vi "HSPA_PSK_TX.vi"() -> ()   [LabVIEW 2025]
doc: "This example shows how simple is to broadcast an Frequency Modulated sound signal using the USRP.\n\n1. Ask the user for a *.wav file.\n2. Read the WAV file.\n3. Select only one channel of the audio data.\n4. Modulate in FM using a frequency deviation of 75kHz. Similar to Radio FM.\n5. Initialize a session.\n6. Configure for arbitrary waveform mode.\n7. Set the output power level and center frequency.\n8. Set the IQ rate to 200k.\n9. Write and read the IQ rate to get the coerced value in order to resample our signal (if needed).\n10. Resample and write the signal to the on board memory. If resample is needed, this step will take little longer depending on the size of the file.\n11. Start the generation.\n12. Check for p the generation.\n13. Stop the generation.\n14. Close the session.\n15. Check for errors."
uses:
  <vilib>/addons/Modulation/Analog/support/mod_Set Error Source.vi
  <vilib>/addons/Modulation/Digital/General/MT Generate PSK System Parameters(M).vi
  Instance           1 28Saved   fm_sound_transmitter .vi
  <vilib>/sound2/lvsound2.llb/Sound File Info (path).vi
  <vilib>/sound2/lvsound2.llb/Sound File Read Open.vi
  <vilib>/addons/Modulation/Digital/Support/Common/Validators/mod_Generate Filter Coefficients Validate.vi
  <vilib>/addons/Modulation/Digital/General/subVIs/mod_Generate Filter Coefficients.vi
  <vilib>/sound2/lvsound2.llb/Sound File Read (DBL).vi
  <vilib>/Waveform/WDTOps.llb/WDT Index Channel DBL.vi
  <instrlib>/niUSRP/niUSRP Write Tx Data (CDB Cluster).vi
  <vilib>/addons/Modulation/niDMT.lvlib
  <vilib>/addons/Modulation/niAMT.lvlib
panel:
  out "sound Chart":waveform(dbl)[](graph)
  out "Frame Size [samples]":i32=4092
  in  "Enabled Channel":string(combo)="0"
  in  "Device Name":refnum<k15>="192.168.10.5"
  in  "filter parameter":dbl=0.5 format="%.2f"
  in  "pulse shaping samples per symbol (16)":i32=16
  in  "pulse shaping filter (none)":T1(ring)
  in  "M":i32=4 min=2 step=2
  in  "Select PSK Modulation Format":T2(tab)=enum."QPSK" caption="PSK"
  in  "QPSK System Parameters":T3={"Samples per Symbol"=8, "symbol map"=[], "Differential PSK"=enum."disable", "PSK type"=0} {"PSK type" items=["normal", "shifted", "offset"]; "symbol map" format="%.3f"}
  in  "pi/4 DQPSK System Parameters":T3={"Samples per Symbol"=8, "symbol map"=[], "Differential PSK"=enum."enable", "PSK type"=1} {"PSK type" items=["normal", "shifted", "offset"]; "symbol map" format="%.3f"}
  in  "OQPSK System Parameters":T3={"Samples per Symbol"=8, "symbol map"=[], "Differential PSK"=enum."disable", "PSK type"=2} {"PSK type" items=["normal", "shifted", "offset"]; "symbol map" format="%.3f"}
  in  "8-PSK System Parameters":T3={"Samples per Symbol"=8, "symbol map"=[], "Differential PSK"=enum."disable", "PSK type"=0} {"PSK type" items=["normal", "shifted", "offset"]; "symbol map" format="%.3f"}
  in  "16-PSK System Parameters":T3={"Samples per Symbol"=8, "symbol map"=[], "Differential PSK"=enum."disable", "PSK type"=0} {"PSK type" items=["normal", "shifted", "offset"]; "symbol map" format="%.3f"}
  in  "Custom System Parameters":T3={"Samples per Symbol"=8, "symbol map"=[], "Differential PSK"=enum."disable", "PSK type"=0} {"PSK type" items=["normal", "shifted", "offset"]; "symbol map" format="%.3f"}
  in  "BPSK System Parameters":T3={"Samples per Symbol"=8, "symbol map"=[], "Differential PSK"=enum."disable", "PSK type"=0} {"PSK type" items=["normal", "shifted", "offset"]; "symbol map" format="%.3f"}
  in  "IQ rate":dbl=100000.0 format="%#_6p"
  out "Constellation Graph 2":T4(graph)
  out "Waveform Graph":waveform(dbl)[](graph)
  in  "Transmitter Gain":dbl format="%.2f"
  in  "frequency (Hz)":dbl=94700000.0 min=500000.0 max=2700000000.0 format="%.2p"
  out "Status":string="Stopped"
  in  "stop":bool
  out "Audio Data":waveform(dbl)[](graph)
  # "USRP Configuration"
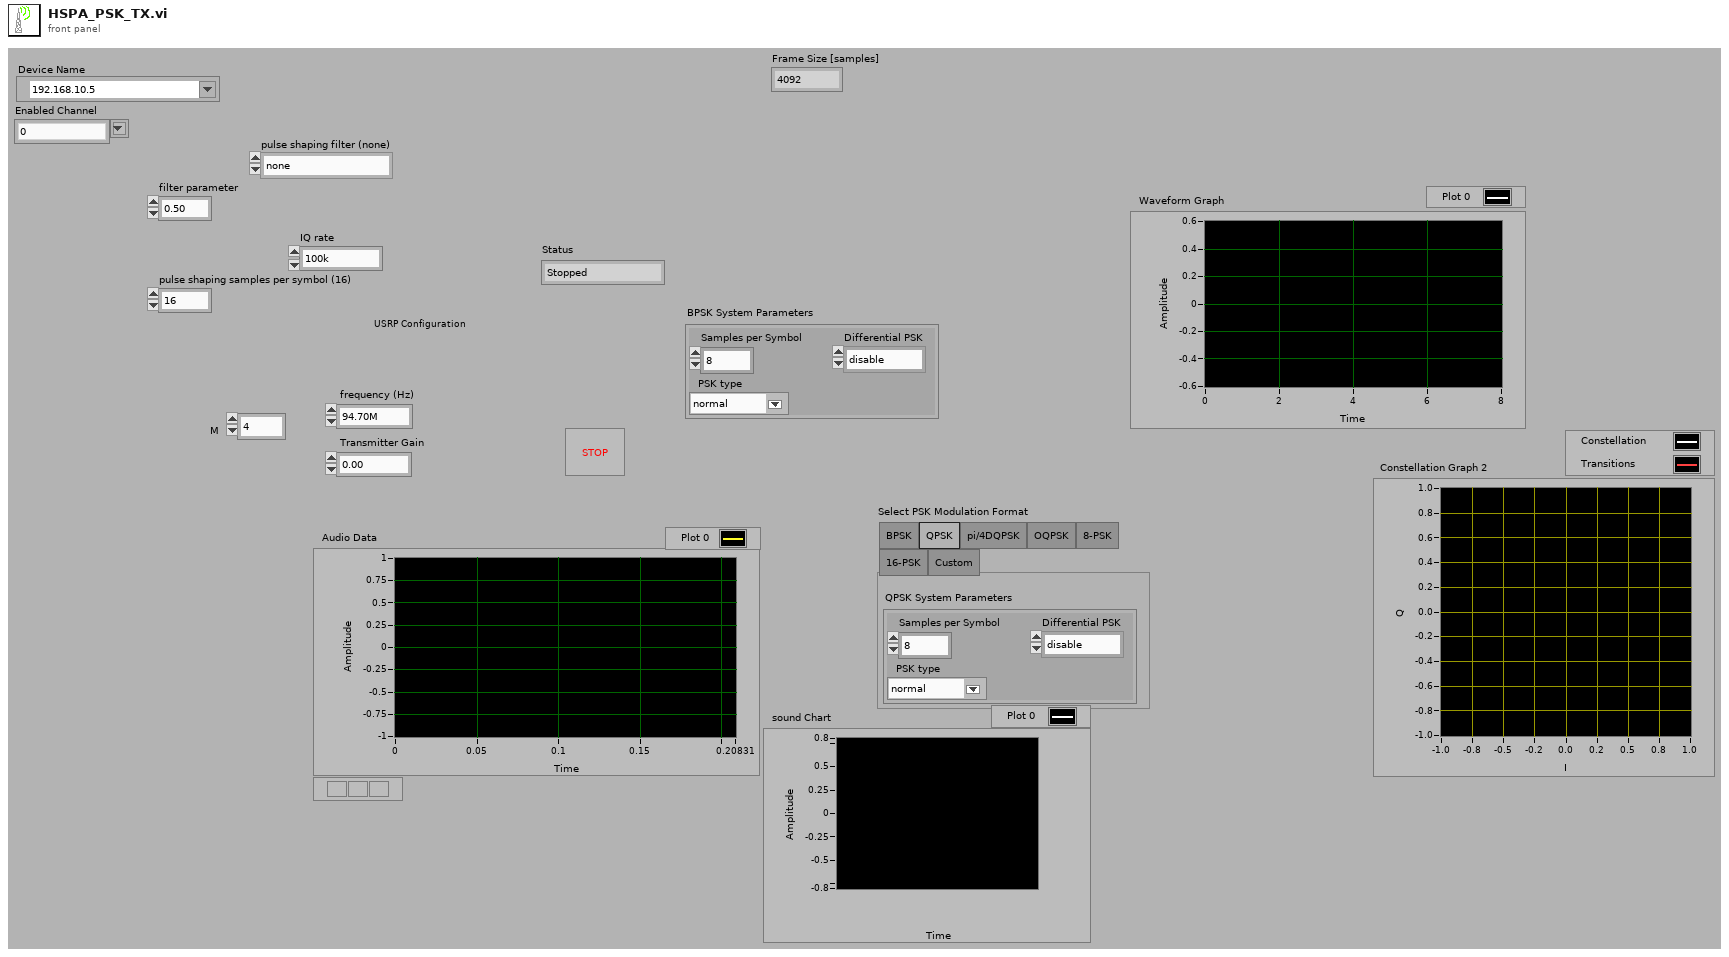
[diagram p1: front panel]
types:
  T1 = enum16{"none", "Raised Cosine", "Root Raised Cos", "Gaussian"}
  T2 = enum32{"BPSK", "QPSK", "pi/4DQPSK", "OQPSK", "8-PSK", "16-PSK", "Custom"}
  T3 = cluster{"Samples per Symbol":i32, "symbol map":cdb[], "Differential PSK":enum16{"disable", "enable"}, "PSK type":u16}
  T4 = cluster{"Decimated Array":dbl[], "Decimated Array":dbl[]}[]
  T5 = cluster{"samples per symbol (16)":i32, "symbol map":cdb[], "differential PSK":enum16{"disable", "enable"}, "PSK type":u16}
  T6 = typedef "Sound File Refnum.ctl" = refnum<file>
  T7 = enum16{"FSK", "PSK", "QAM", "MSK", "PAM", "ASK", "CPM"}
  T8 = typedef "niAMT.lvlib/Complex Data Waveform.ctl" = cluster{"t0":dbl, "dt":dbl, "Y":cdb[]}
  T9 = cluster{"constellation":dbl[], "oversampled data":dbl[]}[]
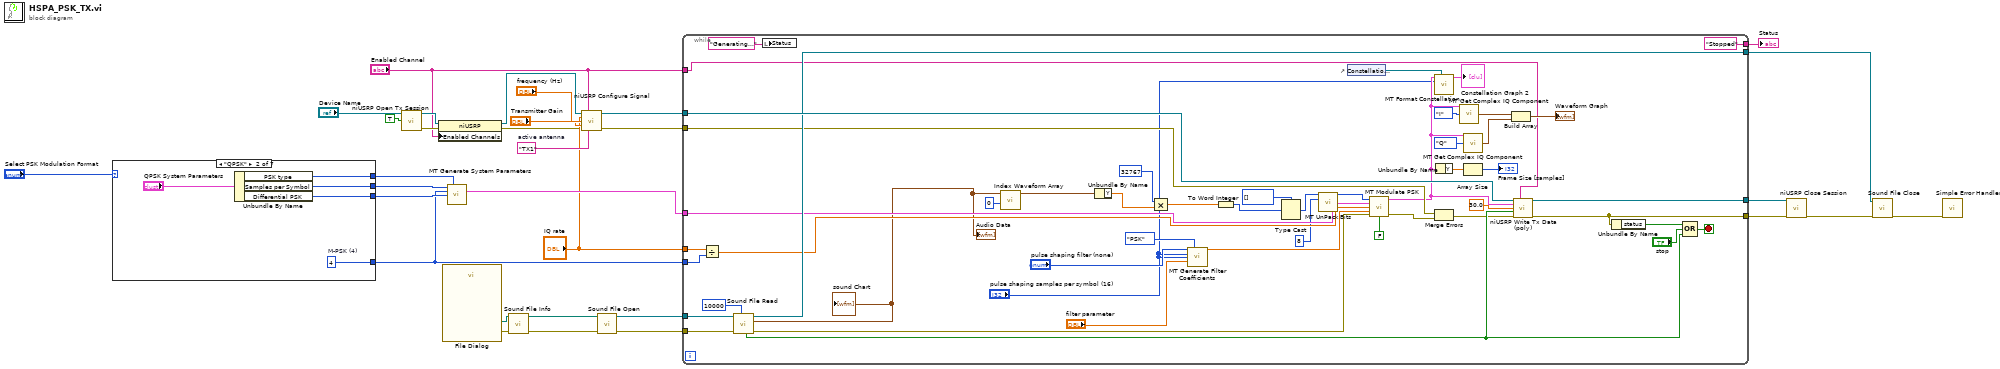
[diagram p0: block diagram]
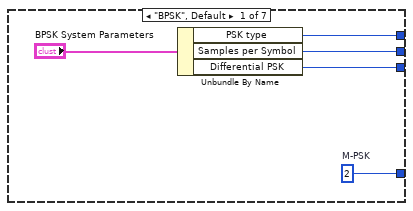
[diagram p2: hidden frame]
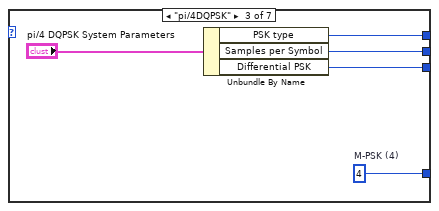
[diagram p3: hidden frame]
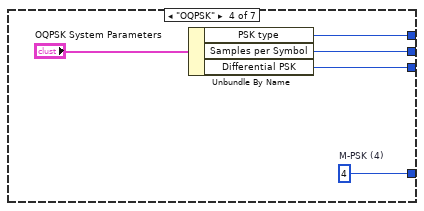
[diagram p4: hidden frame]
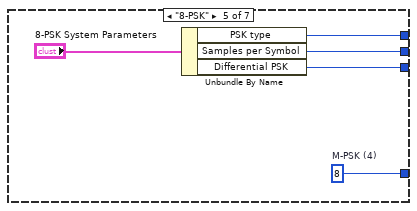
[diagram p5: hidden frame]
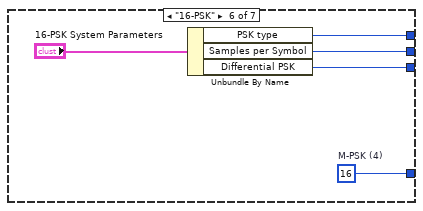
[diagram p6: hidden frame]
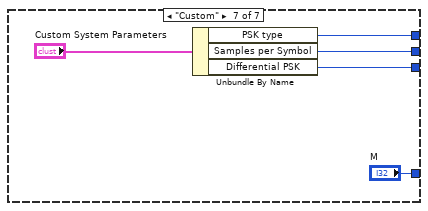
[diagram p7: hidden frame]
diagram:
  w28 = "TX1"  # active antenna
  n1 = case shown="\"QPSK\"" "Select PSK Modulation Format" {
    tunnel: [w33 w38 w45 w50 w55 w61 w64] -> w12
    tunnel: [w34 w39 w44 w49 w54 w60 w65] -> w11
    tunnel: [w36 w41 w46 w51 w53 w59 "M"] -> w8
    tunnel: [w35 w40 w43 w48 w56 w58 w66] -> w13
    frame "BPSK", Default {
      w36 = 2  # M-PSK
      n2 = Unbundle By Name("BPSK System Parameters") -> ("PSK type"=w35:u16, "Samples per Symbol"=w33:i32, "Differential PSK"=w34:enum16{"disable", "enable"})
    }
    frame "QPSK" {
      w41 = 4  # M-PSK (4)
      n3 = Unbundle By Name("QPSK System Parameters") -> ("PSK type"=w40:u16, "Samples per Symbol"=w38:i32, "Differential PSK"=w39:enum16{"disable", "enable"})
    }
    frame "pi/4DQPSK" {
      w46 = 4  # M-PSK (4)
      n4 = Unbundle By Name("pi/4 DQPSK System Parameters") -> ("PSK type"=w43:u16, "Samples per Symbol"=w45:i32, "Differential PSK"=w44:enum16{"disable", "enable"})
    }
    frame "OQPSK" {
      w51 = 4  # M-PSK (4)
      n5 = Unbundle By Name("OQPSK System Parameters") -> ("PSK type"=w48:u16, "Samples per Symbol"=w50:i32, "Differential PSK"=w49:enum16{"disable", "enable"})
    }
    frame "8-PSK" {
      w53 = 8  # M-PSK (4)
      n6 = Unbundle By Name("8-PSK System Parameters") -> ("PSK type"=w56:u16, "Samples per Symbol"=w55:i32, "Differential PSK"=w54:enum16{"disable", "enable"})
    }
    frame "16-PSK" {
      w59 = 16  # M-PSK (4)
      n7 = Unbundle By Name("16-PSK System Parameters") -> ("PSK type"=w58:u16, "Samples per Symbol"=w61:i32, "Differential PSK"=w60:enum16{"disable", "enable"})
    }
    frame "Custom" {
      n8 = Unbundle By Name("Custom System Parameters") -> ("PSK type"=w66:u16, "Samples per Symbol"=w64:i32, "Differential PSK"=w65:enum16{"disable", "enable"})
    }
  }
  n9 = call <instrlib>:"niUSRP Open Tx Session.vi"("device names"="Device Name", "reset"=TRUE) -> ("session handle out"=w5:refnum<k15>, "error out"=w4:errorcluster)  [unwired: 12 in]
  n10 = property class="niUSRP"(reference=w5, error in=w4, "Enabled Channels"="Enabled Channel") -> (reference out=w2:refnum<k15>, error out=w3:errorcluster)
  n11 = call "File Dialog"() -> ("selected path"=w25:path, "error out"=w22:errorcluster)  [unwired: 12 in, 2 out]
  n12 = call-poly <vilib>:"MT Generate System Parameters.vi"("samples per symbol (16)"=w12, "PSK type"=w13, "M-PSK (4)"=w8, "differential PSK"=w11) -> ("PSK system parameters"=w14:T5)  [unwired: 9 in, 2 out]
  n13 = call-poly <vilib>:"Sound File Info.vi"("error in (no error)"=w22, "path"=w25) -> ("error out"=w21:errorcluster, "path out"=w23:path)  [unwired: 6 in, 2 out]
  n14 = call <instrlib>:"niUSRP Configure Signal.vi"("session handle"=w2, "channel list"="Enabled Channel", "IQ rate"="IQ rate", "carrier frequency"="frequency (Hz)", "gain"="Transmitter Gain", "error in (no error)"=w3, "active antenna"=w28) -> ("session handle out"=w27:refnum<k15>, "error out"=w24:errorcluster)  [unwired: 4 in, 3 out]
  n15 = call-poly <vilib>:"Sound File Open.vi"("error in (no error)"=w21, "path"=w23) -> ("error out"=w19:errorcluster, "sound file refnum"=w20:T6)  [unwired: 8 in]
  n16 = while {
    tunnel: ["Stopped" ("Status")] -> w31
    tunnel: w27 -> [w112]
    tunnel: [w111] -> w26
    tunnel: [w110] -> w18
    tunnel: w24 -> [w103]
    tunnel: w20 -> [w107]
    tunnel: w19 -> [w106]
    tunnel: [w105] -> w17
    tunnel: w14 -> [w93]
    tunnel: "IQ rate" -> [w87]
    tunnel: w8 -> [w86]
    tunnel: "Enabled Channel" -> [w85]
    stop <- w114 stop-if-true
    n17 = Divide(x=w87, y=w86) -> (x/y=w88:dbl)
    n18 = call-poly <vilib>:"Sound File Read.vi"("number of samples/ch (-1: all)"=10000, "error in (no error)"=w106, "sound file refnum"=w107) -> ("error out"=w102:errorcluster, "data"=w68:waveform(dbl)[], "sound file refnum out"=w105:T6, "end of file?"=w108:bool)  [unwired: 4 in, 1 out]
    "Audio Data" <- w68
    "sound Chart" <- w68
    n19 = local write "Status"("Generating..." ("Status")) -> ()
    n20 = call-poly <vilib>:"Index Waveform Array.vi"("index"=0, "waveform array"=w68) -> ("waveform"=w73:waveform(dbl))  [unwired: 8 in, 1 out]
    n21 = Unbundle By Name(w73) -> ("Y"=w72:dbl[])
    n22 = Multiply(x=32767, y=w72) -> (x*y=w77:dbl[])
    n23 = call <vilib>:"MT Generate Filter Coefficients.vi"("pulse shaping filter (none)"="pulse shaping filter (none)", "modulation type"=T7."PSK", "pulse shaping samples per symbol (16)"="pulse shaping samples per symbol (16)", "matched samples per symbol (16)"="pulse shaping samples per symbol (16)", "filter parameter"="filter parameter") -> ("pulse shaping filter coefficients"=w89:dbl[])  [unwired: 8 in, 2 out]
    n24 = To Word Integer(number=w77) -> (16bit integer=w76:i16[])
    n25 = Type Cast(type=u8[] [], x=w76) -> (*(type *) &x=w71:u8[])
    n26 = call <vilib>:"MT UnPack Bits.vi"("input integers"=w71, "bits per integer"=8) -> ("output bit stream"=w70:i8[])  [unwired: 12 in, 1 out]
    n27 = control-ref of="Constellation Graph 2"() -> (w99:refnum<vi>)
    n28 = call <vilib>:"MT Modulate PSK.vi"("input bit stream"=w70, "PSK system parameters"=w93, "symbol rate (Hz)"=w88, "pulse shaping filter coefficients"=w89, "error in (no error)"=w102, "reset? (T)"=FALSE) -> ("output complex waveform"=w81:T8, "error out"=w101:errorcluster)  [unwired: 7 in, 1 out]
    n29 = call <vilib>:"MT Format Constellation.vi"("waveform"=w81, "constellation reference"=w99, "samples per symbol"="pulse shaping samples per symbol (16)") -> ("constellation graph"=→"Constellation Graph 2":T9)  [unwired: 2 in, 10 out]
    n30 = Merge Errors(w103, w101) -> (w104:errorcluster)
    n31 = Unbundle By Name(w81) -> ("Y"=w83:cdb[])
    n32 = call <vilib>:"MT Get Complex IQ Component.vi"("IQ data (complex) in"=w81, "component choice"=enum16{"I", "Q", "Magnitude", "Phase"}."I") -> ("CE component"=w96:waveform(dbl))  [unwired: 11 in, 2 out]
    n33 = call <vilib>:"MT Get Complex IQ Component.vi"("IQ data (complex) in"=w81, "component choice"=enum16{"I", "Q", "Magnitude", "Phase"}."Q") -> ("CE component"=w97:waveform(dbl))  [unwired: 11 in, 2 out]
    n34 = Array Size(array=w83) -> (size(s)=→"Frame Size [samples]":i32)
    n35 = Build Array(w96, w97) -> (→"Waveform Graph":waveform(dbl)[])
    n36 = call-poly <instrlib>:"niUSRP Write Tx Data (poly).vi"("session handle"=w112, "channel list"=w85, "data"=w81, "timeout"=30.0, "end of data?"=w108, "error in (no error)"=w104) -> ("session handle out"=w111:refnum<k15>, "error out"=w110:errorcluster)  [unwired: 8 in]
    n37 = Unbundle By Name(w110) -> ("status"=w109:bool)
    n38 = Compound Arithmetic op=OR(w109, "stop", w108) -> (w114:bool)
  }
  "Status" <- w31
  n39 = call <instrlib>:"niUSRP Close Session.vi"("session handle"=w26, "error in (no error)"=w18) -> ("error out"=w15:errorcluster)  [unwired: 13 in]
  n40 = call <vilib>:"Sound File Close.vi"("error in (no error)"=w15, "sound file refnum"=w17) -> ("error out"=w16:errorcluster)  [unwired: 9 in]
  n41 = call <vilib>:"Simple Error Handler.vi"("error in (no error)"=w16) -> ()  [unwired: 4 in, 5 out]
